vi "Read Steps.vi"(8 "error in (no error)":errorcluster, 11 "SequenceIndex in":refnum<class "SequenceIndex.lvclass">) -> (0 "error out":errorcluster, 2 "Steps":u32=1, 3 "SequenceIndex out":refnum<class "SequenceIndex.lvclass">)   [LabVIEW 2013, in "SequenceIndex.lvclass"]
uses:
  SequenceIndex.lvclass
  SequenceIndex.lvclass/SequenceIndex.ctl
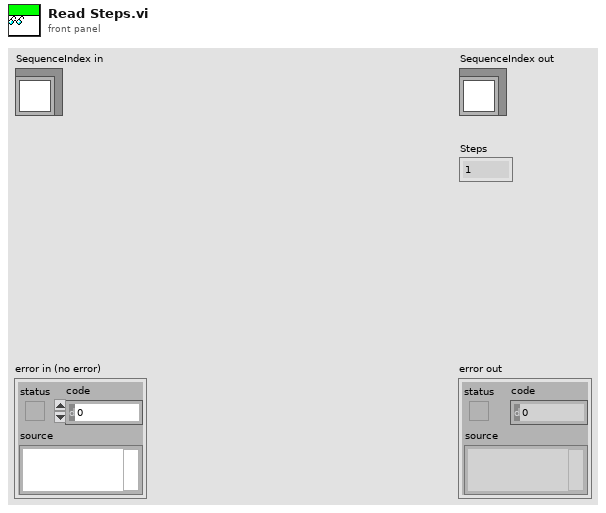
[diagram p1: front panel]
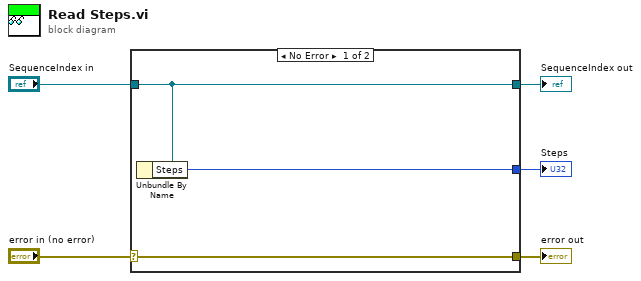
[diagram p0: block diagram]
diagram:
  n1 = case shown="No Error" "error in (no error)" {
    selector: "error in (no error)" -> [w8 w9]
    tunnel: [w8 w9] -> w4
    tunnel: [w7 w10] -> w2
    tunnel: "SequenceIndex in" -> [w7 w10]
    tunnel: [w6 _] -> w1
    frame No Error {
      n2 = Unbundle By Name(w7) -> ("Steps"=w6:u32)
    }
    frame Error {
    }
  }
  "error out" <- w4
  "SequenceIndex out" <- w2
  "Steps" <- w1
